vi "ABB Select Heat run.vi"() -> (2 "Measure out":enum16{"Full Load", "Partial Load", "No Load"}(ring), 3 "Heat run Type out":enum16{"Full Load", "Partial- & No-Load"}(ring))   [LabVIEW 2017]
uses:
  ABB global.vi
panel:
  in  "Next":bool
  in  "Measure":enum16{"Full Load", "Partial Load", "No Load"}(ring)
  in  "Heat run Type":enum16{"Full Load", "Partial- & No-Load"}(ring)
  # "SELECT HEAT RUN"
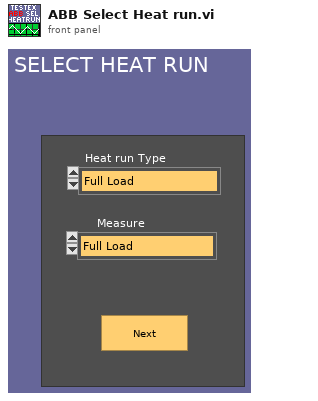
[diagram p1: front panel]
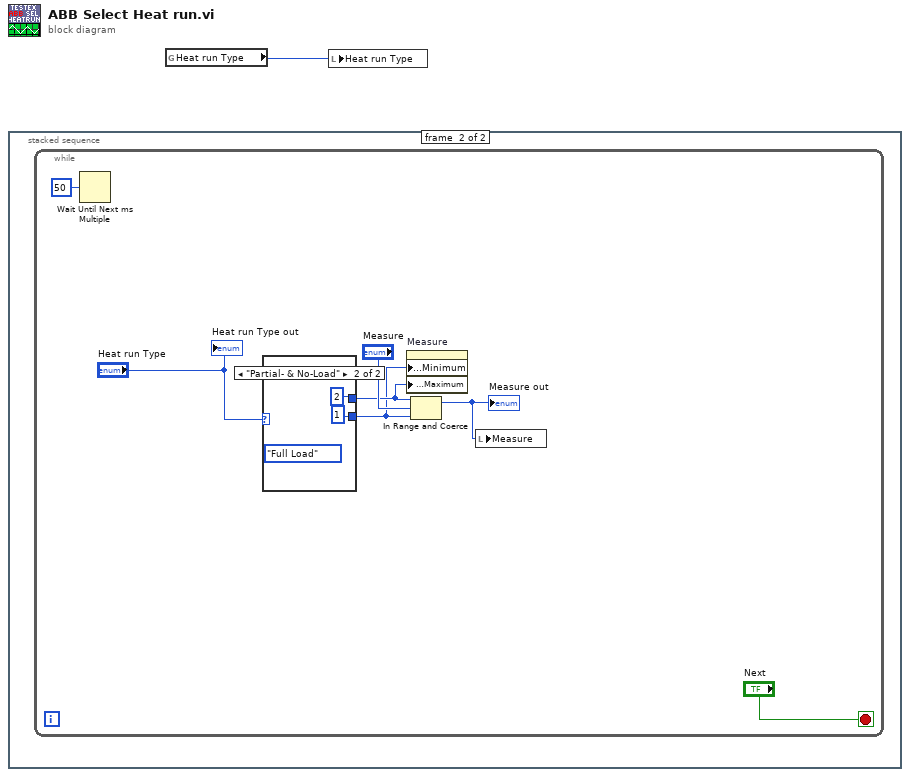
[diagram p0: block diagram]
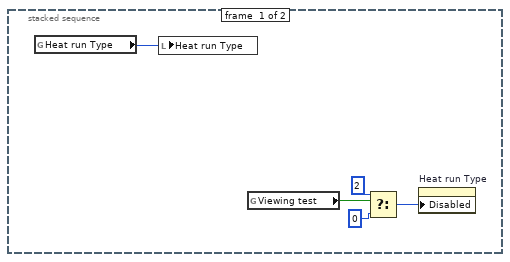
[diagram p2: hidden frame]
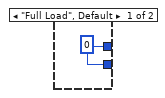
[diagram p3: hidden frame]
diagram:
  n1 = stacked-sequence {
    frame #0 {
      n2 = global read "ABB global.vi" "Heat run Type"() -> (w3:enum16{"Full Load", "Partial- & No-Load"})
      n3 = local write "Heat run Type"(w3) -> ()
      n4 = global read "ABB global.vi" "Viewing test"() -> (w6:bool)
      n5 = Select(t=2, s=w6, f=0) -> (s? t:f=w2:i32)
      n6 = property on="Heat run Type" class="Enum (strict)"("Disabled"=w2) -> ()  [unwired: 2 in, 2 out]
    }
    frame #1 {
      n7 = while {
        stop <- "Next" stop-if-true
        n8 = Wait Until Next ms Multiple(millisecond multiple=u32 50) -> ()  [unwired: 1 out]
        n9 = case shown="\"Partial- & No-Load\"" "Heat run Type" {
          tunnel: [w14 1] -> w7
          tunnel: [w14 2] -> w8
          frame "Full Load", Default {
            w14 = 0
          }
          frame "Partial- & No-Load" {
            (unwired) enum16{"Full Load", "Partial- & No-Load"}."Full Load" ("Heat run Type")
          }
        }
        n10 = property on="Measure" class="Enum (strict)"("Data Entry Limits:Minimum"=w7, "Data Entry Limits:Maximum"=w8) -> ()  [unwired: 2 in, 2 out]
        n11 = In Range and Coerce(upper limit=w8, x="Measure", lower limit=w7) -> (coerced(x)=w9:i32)  [unwired: 1 out]
        "Measure out" <- w9
        n12 = local write "Measure"(w9) -> ()
        "Heat run Type out" <- "Heat run Type"
      }
    }
  }
  n13 = global read "ABB global.vi" "Heat run Type"() -> (w1:enum16{"Full Load", "Partial- & No-Load"})
  n14 = local write "Heat run Type"(w1) -> ()
